vi "Facade.vi"(0 "Data In":T5, 2 "Display State In":T2, 3 "Container State":T4) -> (6 "Data Out":T5, 7 "Display State Out":T2, 8 "Action":T1)   [LabVIEW 2017, in "XY Plot Matrix.xctl"]
uses:
  <vilib>/Math Plots/2D Math Plots/XY Plot Matrix/XY Plot Matrix XCtrl/XY Plot Matrix.xctl
  <vilib>/Math Plots/2D Math Plots/XY Plot Matrix/XY Plot Matrix XCtrl/Data.ctl
  <vilib>/Math Plots/2D Math Plots/XY Plot Matrix/XY Plot Matrix Datatype/XY Plot Matrix Datatype.lvclass
  <vilib>/_xctls/Container State.ctl
  <vilib>/Math Plots/2D Math Plots/XY Plot Matrix/XY Plot Matrix XCtrl/State.ctl
  <vilib>/Math Plots/2D Math Plots/XY Plot Matrix/XY Plot Matrix/XY Plot Matrix.lvclass
  <vilib>/Math Plots/2D Math Plots/2D Plot/Action String/XYPlotMatrix Ctrl Act Queue.ctl
  <vilib>/Math Plots/2D Math Plots/2D Plot/Action String/XYPlotMatrix Ctrl Act Cluster.ctl
  <vilib>/Math Plots/2D Math Plots/2D Plot/Action String/2DMathPlot State Class.ctl
  <vilib>/_xctls/Action.ctl
  <vilib>/Math Plots/2D Math Plots/2D Plot/Action String/2DMathPlot Action String.ctl
  <vilib>/_xctls/XControlSupport.lvlib
  <vilib>/Math Plots/Plot Private Lib/NI_Math Plot Private Lib.lvlib
panel:
  out "Export Image":picture
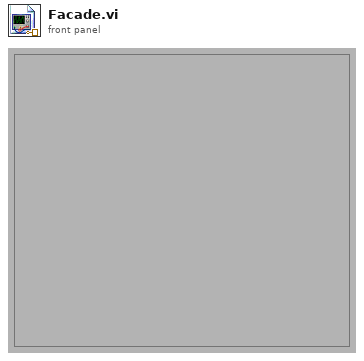
[diagram p1: front panel]
types:
  T1 = typedef "XControlSupport.lvlib/Action.ctl" = cluster{"Data Changed?":bool, "State Changed?":bool, "Action Name":string}
  T2 = typedef "XY Plot Matrix.xctl/State.ctl" = cluster{"XY Plot Matrix.lvclass":refnum<class "XY Plot Matrix.lvclass">, "Control Ref Queue":T3, "Main Frame Color":u32}
  T3 = typedef "XYPlotMatrix Ctrl Act Queue.ctl" = refnum<queue>
  T4 = typedef "XControlSupport.lvlib/Container State.ctl" = cluster{"Indicator?":bool, "Run Mode?":bool, " Refnum":refnum<vi>}
  T5 = typedef "XY Plot Matrix.xctl/Data.ctl" = refnum<class "XY Plot Matrix Datatype.lvclass">[]
  T6 = typedef "XYPlotMatrix Ctrl Act Cluster.ctl" = cluster{"Facade VI":refnum<vi>, "XControl":refnum<vi>, "Sub Panel":refnum<vi>, "Sub VI":refnum<vi>, "Export Image":refnum<vi>, "Display State Change Class":T7}
  T7 = typedef "2DMathPlot State Class.ctl" = enum16{"Update All (Undo)", "Update General", "Update Appearance", "Update Format", "Update Scale", "Update Marker", "Update Cursor", "None"}
  T8 = typedef "XY Plot Matrix.lvclass/Mulitmatrix Representation.ctl" = cluster{"Matrix Representation Array":T9[][], "Max Range Array":T10[][], "Max Plot Number":i32}
  T9 = typedef "XY Plot Matrix.lvclass/Matrix Representation.ctl" = cluster{"Graph Matrix":cluster{"X":dbl[], "Y":dbl[]}[]}
  T10 = typedef "2D Plot.lvclass/Range Cluster.ctl" = cluster{"X Range":cluster{"Max X":dbl, "Min X":dbl}, "Y Range":cluster{"Max Y":dbl, "Min Y":dbl}}
  T11 = typedef "2DMathPlot Action String.ctl" = u16
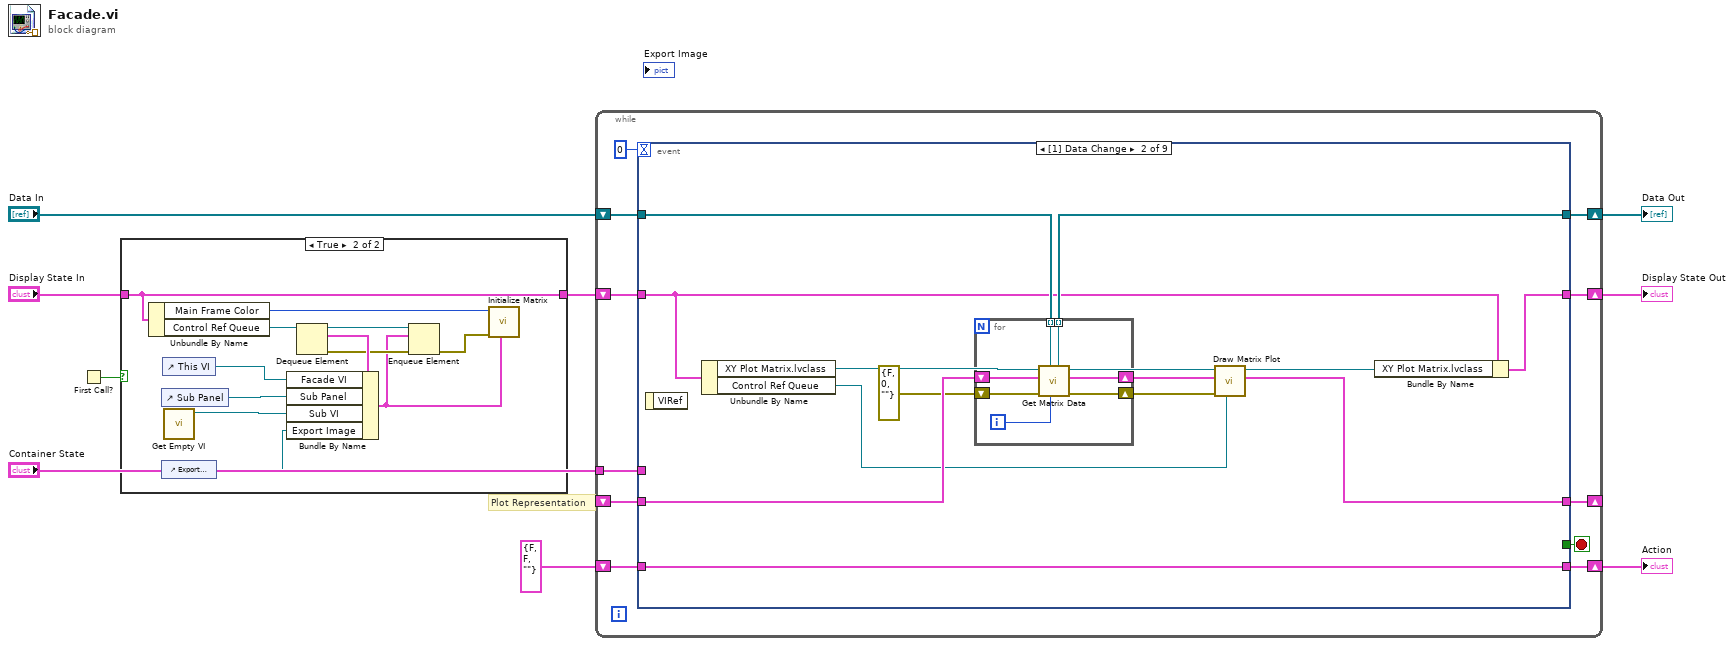
[diagram p0: block diagram]
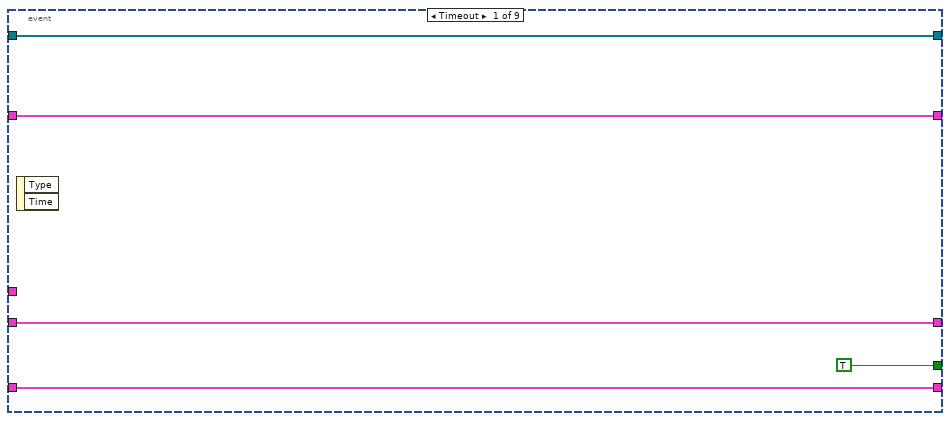
[diagram p3: hidden frame]
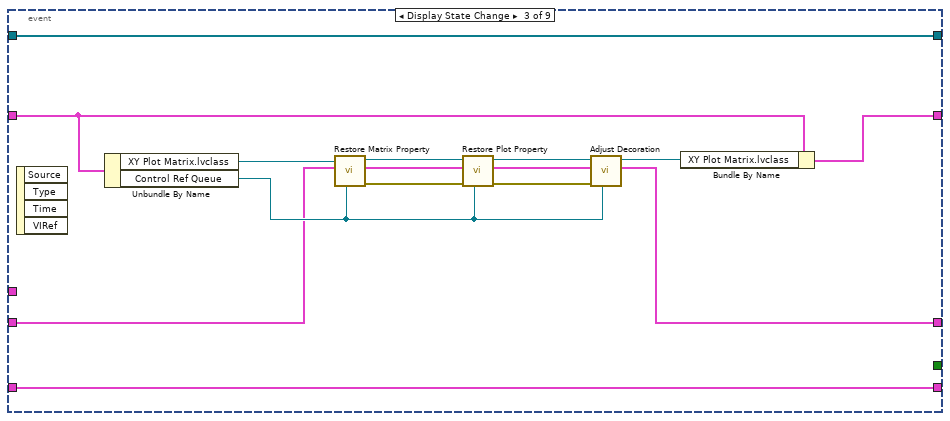
[diagram p4: hidden frame]
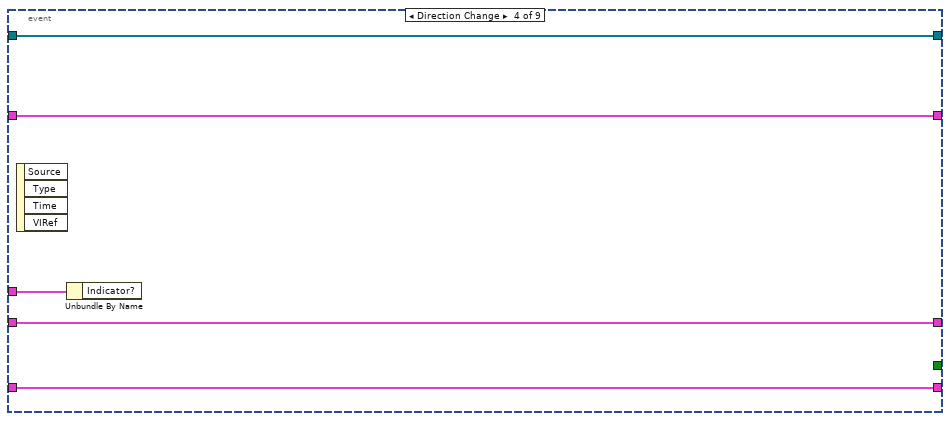
[diagram p5: hidden frame]
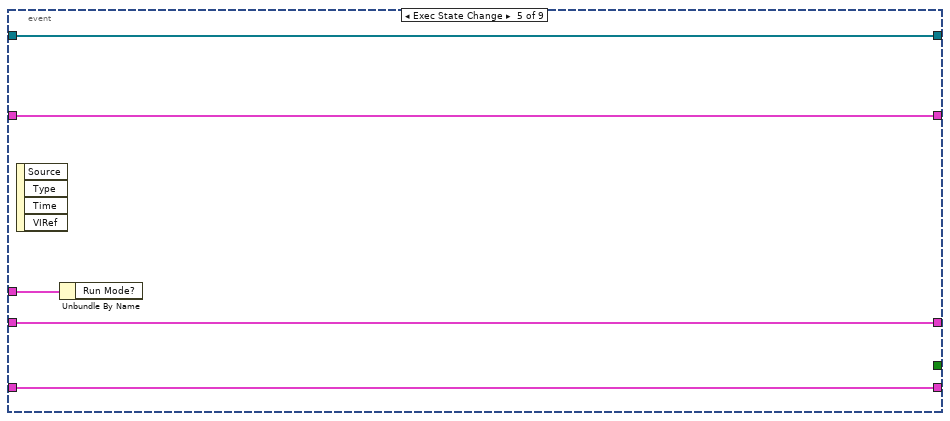
[diagram p6: hidden frame]
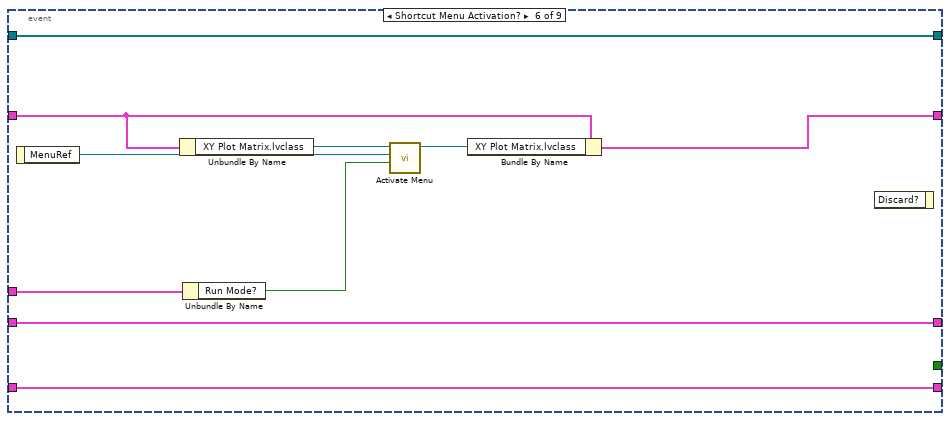
[diagram p7: hidden frame]
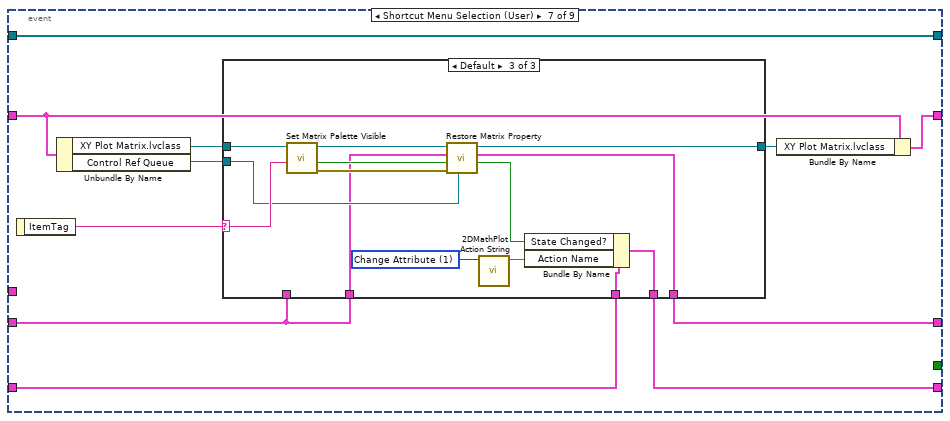
[diagram p8: hidden frame]
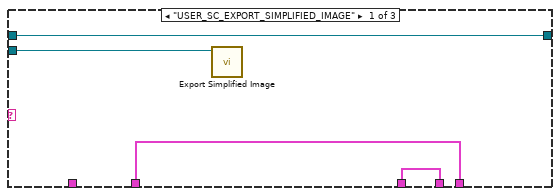
[diagram p9: hidden frame]
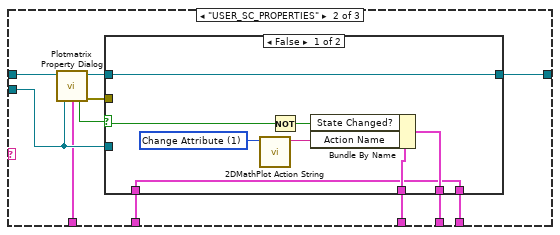
[diagram p10: hidden frame]
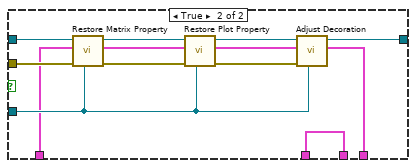
[diagram p11: hidden frame]
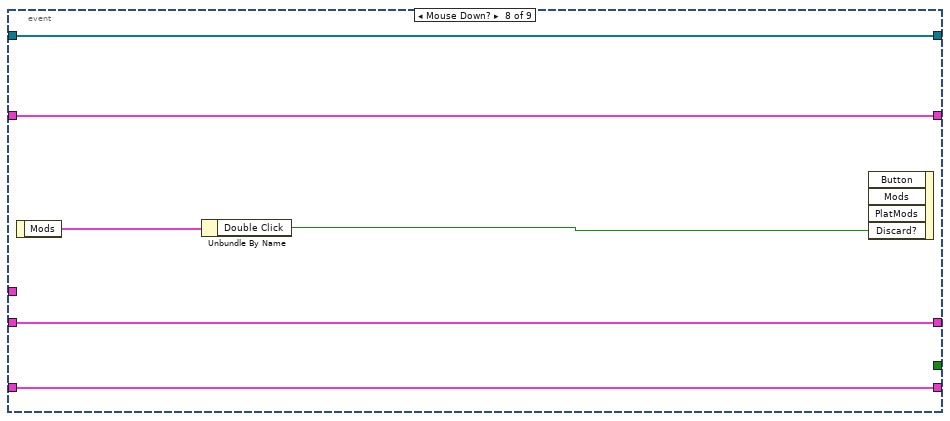
[diagram p12: hidden frame]
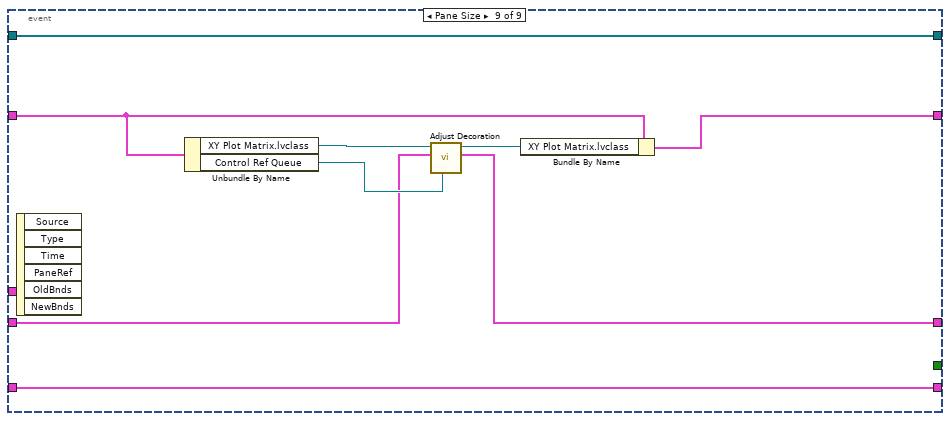
[diagram p13: hidden frame]
diagram:
  # "Plot Representation"
  n1 = First Call?() -> (First Call?: T/F=w3:bool)
  n2 = case shown="True" w3 {
    tunnel: "Display State In" -> [w10 w19]
    tunnel: [w10 w19] -> w1
    frame False {
    }
    frame True {
      n3 = Unbundle By Name(w19) -> ("Main Frame Color"=w11:u32, "Control Ref Queue"=w21:T3)
      n4 = control-ref of="Sub Panel"() -> (w16:refnum<vi>)
      n5 = control-ref of="Export Image"() -> (w12:refnum<vi>)
      n6 = control-ref of="This VI"() -> (w18:refnum<vi>)
      n7 = call <vilib>:"Get Empty VI.vi"() -> ("vi refnum"=w17:refnum<vi>)  [unwired: 11 out]
      n8 = Dequeue Element(queue=w21) -> (queue out=w22:T3, element=w20:T6, error out=w14:errorcluster)  [unwired: 1 in, 2 out]
      n9 = Bundle By Name(cluster=w20, "Facade VI"=w18, "Sub Panel"=w16, "Sub VI"=w17, "Export Image"=w12) -> (w13:T6)
      n10 = Enqueue Element(queue=w22, element=w13, error in (no error)=w14) -> (error out=w15:errorcluster)  [unwired: 3 out]
      n11 = call <vilib>:"Initialize Matrix.vi"("Control Ref Cluster"=w13, "error in (no error)"=w15, "Main Frame Color"=w11) -> ()  [unwired: 9 out]
    }
  }
  n12 = while {
    shift-right: [w32] -> w6
    shift-left: w1 -> [w33]
    tunnel: "Container State" -> [w29]
    shift-right: [w27] -> w9
    shift-left: "Data In" -> [w28]
    shift-right: [w25] -> w5
    shift-left: T1 {"Data Changed?"=FALSE, "State Changed?"=FALSE, "Action Name"=""} ("Action") -> [w26]
    shift-right: [w23] -> _
    shift-left: _ -> [w24]
    stop <- w31 stop-if-true
    n13 = event shown="[1] Data Change" {
      selector: _ -> [_ _ _ _ _ _ _ _ _]
      dyn-events: _ -> [_ _ _ _ _ _ _ _ _]
      timeout: 0 -> [_ _ _ _ _ _ _ _ _]
      tunnel: w33 -> [w34 w42 w69 w76 w81 w86 w102 w154 w161]
      tunnel: [w34 w41 w68 w76 w81 w85 w101 w154 w160] -> w32
      tunnel: [TRUE _ _ _ _ _ _ _ _] -> w31
      tunnel: w29 -> [_ _ _ w77 w82 w88 _ _ _]
      tunnel: w28 -> [w36 w50 w72 w75 w80 w90 w103 w155 w164]
      tunnel: [w36 w49 w72 w75 w80 w90 w103 w155 w164] -> w27
      tunnel: [w37 w51 w71 w74 w79 w92 w97 w152 w166] -> w25
      tunnel: w26 -> [w37 w51 w71 w74 w79 w92 w95 w152 w166]
      tunnel: w24 -> [w35 w48 w60 w73 w78 w91 w93 w153 w159]
      tunnel: [w35 w46 w61 w73 w78 w91 w94 w153 w158] -> w23
      event Timeout {
        n14 = event-data() -> ()  [unwired: 3 out]
      }
      event Data Change {
        n15 = event-data() -> ()  [unwired: 2 out]
        n16 = Unbundle By Name(w42) -> ("XY Plot Matrix.lvclass"=w43:refnum<class "XY Plot Matrix.lvclass">, "Control Ref Queue"=w40:T3)
        n17 = for {
          tunnel: w50 -> [w58] mode=indexing
          tunnel: [w57] -> w49 mode=indexing
          shift-right: [w56] -> w47
          shift-left: w48 -> [w55]
          shift-right: [w53] -> w45
          shift-left: errorcluster {"status"=FALSE, "code"=0, "source"=""} ("error out") -> [w52]
          i -> [w54]
          n18 = call <vilib>:"Get Matrix Data.vi"("Index"=w54, "2D Plotmatrix Datatype.lvclass in"=w58, "error in (no error)"=w52, "Matrix Representation Array In"=w55) -> ("error out"=w53:errorcluster, "Matrix Representation Array Out"=w56:T8, "2D Plotmatrix Datatype.lvclass out"=w57:refnum<class "XY Plot Matrix Datatype.lvclass">)  [unwired: 5 out]
        }
        n19 = call <vilib>:"Draw Matrix Plot.vi"("Control Ref Queue"=w40, "error in (no error)"=w45, "Matrix Representation Array In"=w47, "2D Plotmatrix.lvclass in"=w43) -> ("Matrix Representation Array Out"=w46:T8, "2D Plotmatrix.lvclass out"=w39:refnum<class "XY Plot Matrix.lvclass">)  [unwired: 6 out]
        n20 = Bundle By Name(cluster=w42, "XY Plot Matrix.lvclass"=w39) -> (w41:T2)
      }
      event Display State Change {
        n21 = event-data() -> ()  [unwired: 5 out]
        n22 = Unbundle By Name(w69) -> ("XY Plot Matrix.lvclass"=w70:refnum<class "XY Plot Matrix.lvclass">, "Control Ref Queue"=w65:T3)
        n23 = call <vilib>:"Restore Matrix Property.vi"("Control Ref Queue"=w65, "Matrix Representation Array In"=w60, "2D Plotmatrix.lvclass in"=w70) -> ("error out"=w66:errorcluster, "Matrix Representation Array Out"=w59:T8, "2D Plotmatrix.lvclass out"=w67:refnum<class "XY Plot Matrix.lvclass">)  [unwired: 1 in, 5 out]
        n24 = call <vilib>:"Restore Plot Property.vi"("Control Ref Queue"=w65, "error in (no error)"=w66, "2D Plotmatrix.lvclass in"=w67) -> ("error out"=w64:errorcluster, "2D Plotmatrix.lvclass out"=w63:refnum<class "XY Plot Matrix.lvclass">)  [unwired: 7 out]
        n25 = call <vilib>:"Adjust Decoration.vi"("Control Ref Queue"=w65, "error in (no error)"=w64, "Matrix Representation Array In"=w59, "2D Plotmatrix.lvclass in"=w63) -> ("Matrix Representation Array Out"=w61:T8, "2D Plotmatrix.lvclass out"=w62:refnum<class "XY Plot Matrix.lvclass">)  [unwired: 6 out]
        n26 = Bundle By Name(cluster=w69, "XY Plot Matrix.lvclass"=w62) -> (w68:T2)
      }
      event Direction Change {
        n27 = event-data() -> ()  [unwired: 5 out]
        n28 = Unbundle By Name(w77) -> ()  [unwired: 1 out]
      }
      event Exec State Change {
        n29 = event-data() -> ()  [unwired: 5 out]
        n30 = Unbundle By Name(w82) -> ()  [unwired: 1 out]
      }
      event Shortcut Menu Activation? {
        n31 = event-data() -> ("MenuRef"=w89:refnum<k9>)  [unwired: 1 out]
        n32 = Unbundle By Name(w86) -> ("XY Plot Matrix.lvclass"=w84:refnum<class "XY Plot Matrix.lvclass">)
        n33 = Unbundle By Name(w88) -> ("Run Mode?"=w87:bool)
        n34 = call-dynamic "Activate Menu.vi"("Run mode?"=w87, "MenuRef"=w89, "2D Plotmatrix.lvclass in"=w84) -> ("2D Plotmatrix.lvclass out"=w83:refnum<class "XY Plot Matrix.lvclass">)  [unwired: 1 in, 7 out]
        n35 = Bundle By Name(cluster=w86, "XY Plot Matrix.lvclass"=w83) -> (w85:T2)
        n36 = event-data() -> ()  [unwired: 1 in, 2 out]
      }
      event Shortcut Menu Selection (User) {
        n37 = event-data() -> ("ItemTag"=w96:string)  [unwired: 1 out]
        n38 = Unbundle By Name(w102) -> ("XY Plot Matrix.lvclass"=w100:refnum<class "XY Plot Matrix.lvclass">, "Control Ref Queue"=w98:T3)
        n39 = case shown="Default" w96 {
          selector: w96 -> [_ _ w146]
          tunnel: w100 -> [w106 w118 w151]
          tunnel: [w106 w114 w144] -> w99
          tunnel: w98 -> [w107 w112 w143]
          tunnel: [w105 w115 w147] -> w97
          tunnel: w95 -> [w105 w116 w141]
          tunnel: w93 -> [w104 w110 w140]
          tunnel: [w104 w109 w139] -> w94
          tunnel: w93 -> [_ w108 _]
          frame "USER_SC_EXPORT_SIMPLIFIED_IMAGE" {
            n40 = call <vilib>:"Export Simplified Image.vi"("Control Ref Queue"=w107) -> ()  [unwired: 11 out]
          }
          frame "USER_SC_PROPERTIES" {
            n41 = call <vilib>:"Plotmatrix Property Dialog.vi"("Control Ref Queue"=w112, "Multimatrix Representation"=w108, "2D Feather.lvclass in"=w118) -> ("error out"=w111:errorcluster, "2D Feather.lvclass out"=w113:refnum<class "XY Plot Matrix.lvclass">, "Cancel?"=w117:bool)  [unwired: 1 in, 5 out]
            n42 = case shown="False" w117 {
              selector: w117 -> [w123 _]
              tunnel: w116 -> [w122 w138]
              tunnel: [w121 w138] -> w115
              tunnel: [w120 w130] -> w114
              tunnel: w113 -> [w120 w135]
              tunnel: w112 -> [_ w132]
              tunnel: w111 -> [_ w134]
              tunnel: w110 -> [w119 w128]
              tunnel: [w119 w129] -> w109
              frame False {
                w126 = T11 1 items=["Show/Hide", "Change Attribute", "Text Edit", "Cursor Move"] ("Global String")
                n43 = call <vilib>:"2DMathPlot Action String.vi"("Global String"=w126) -> ("String Out"=w125:string)  [unwired: 10 out]
                n44 = Not(x=w123) -> (.not. x?=w124:bool)
                n45 = Bundle By Name(cluster=w122, "State Changed?"=w124, "Action Name"=w125) -> (w121:T1)
              }
              frame True {
                n46 = call <vilib>:"Restore Matrix Property.vi"("Control Ref Queue"=w132, "error in (no error)"=w134, "Matrix Representation Array In"=w128, "2D Plotmatrix.lvclass in"=w135) -> ("error out"=w136:errorcluster, "Matrix Representation Array Out"=w127:T8, "2D Plotmatrix.lvclass out"=w137:refnum<class "XY Plot Matrix.lvclass">)  [unwired: 5 out]
                n47 = call <vilib>:"Restore Plot Property.vi"("Control Ref Queue"=w132, "error in (no error)"=w136, "2D Plotmatrix.lvclass in"=w137) -> ("error out"=w133:errorcluster, "2D Plotmatrix.lvclass out"=w131:refnum<class "XY Plot Matrix.lvclass">)  [unwired: 7 out]
                n48 = call <vilib>:"Adjust Decoration.vi"("Control Ref Queue"=w132, "error in (no error)"=w133, "Matrix Representation Array In"=w127, "2D Plotmatrix.lvclass in"=w131) -> ("Matrix Representation Array Out"=w129:T8, "2D Plotmatrix.lvclass out"=w130:refnum<class "XY Plot Matrix.lvclass">)  [unwired: 6 out]
              }
            }
          }
          frame Default {
            w149 = T11 1 items=["Show/Hide", "Change Attribute", "Text Edit", "Cursor Move"] ("Global String")
            n49 = call <vilib>:"Set Matrix Palette Visible.vi"("Item Tag"=w146, "2D Plotmatrix in"=w151) -> ("error out"=w142:errorcluster, "State Change?"=w148:bool, "2D Plotmatrix out"=w145:refnum<class "XY Plot Matrix.lvclass">)  [unwired: 2 in, 5 out]
            n50 = call <vilib>:"Restore Matrix Property.vi"("Control Ref Queue"=w143, "error in (no error)"=w142, "Matrix Representation Array In"=w140, "2D Plotmatrix.lvclass in"=w145) -> ("Matrix Representation Array Out"=w139:T8, "2D Plotmatrix.lvclass out"=w144:refnum<class "XY Plot Matrix.lvclass">)  [unwired: 6 out]
            n51 = call <vilib>:"2DMathPlot Action String.vi"("Global String"=w149) -> ("String Out"=w150:string)  [unwired: 10 out]
            n52 = Bundle By Name(cluster=w141, "State Changed?"=w148, "Action Name"=w150) -> (w147:T1)
          }
        }
        n53 = Bundle By Name(cluster=w102, "XY Plot Matrix.lvclass"=w99) -> (w101:T2)
      }
      event Mouse Down? {
        n54 = event-data() -> ("Mods"=w157:cluster{"Double Click":bool, "Menu Key":bool})  [unwired: 1 out]
        n55 = Unbundle By Name(w157) -> ("Double Click"=w156:bool)
        n56 = event-data("Discard?"=w156) -> ()  [unwired: 1 in, 4 out]
      }
      event Pane Size {
        n57 = event-data() -> ()  [unwired: 7 out]
        n58 = Unbundle By Name(w161) -> ("XY Plot Matrix.lvclass"=w163:refnum<class "XY Plot Matrix.lvclass">, "Control Ref Queue"=w165:T3)
        n59 = call <vilib>:"Adjust Decoration.vi"("Control Ref Queue"=w165, "Matrix Representation Array In"=w159, "2D Plotmatrix.lvclass in"=w163) -> ("Matrix Representation Array Out"=w158:T8, "2D Plotmatrix.lvclass out"=w162:refnum<class "XY Plot Matrix.lvclass">)  [unwired: 1 in, 6 out]
        n60 = Bundle By Name(cluster=w161, "XY Plot Matrix.lvclass"=w162) -> (w160:T2)
      }
    }
  }
  "Display State Out" <- w6
  "Data Out" <- w9
  "Action" <- w5
